vi "Initialization VI.vi"(8 "error in (no error)":errorcluster, 10 "Custom XML":string, 11 "Device Item Ref in":T1 format="%.0x") -> (0 "error out":errorcluster, 3 "Device Item Ref out":T1 format="%.0x")   [LabVIEW 2023, in "NI 272x Resistive Simulation Custom Device Configuration.lvlib"]
uses:
  NI 272x Resistive Simulation Custom Device Configuration.lvlib
  <vilib>/NI VeriStand/Custom Device API/Custom Device Item Ref.ctl
  <vilib>/NI VeriStand/Custom Device API/Custom Device Loop Type.ctl
  <vilib>/NI VeriStand/Custom Device API/Custom Device API.lvlib
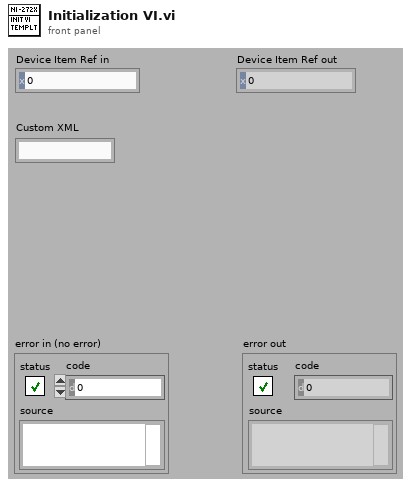
[diagram p1: front panel]
types:
  T1 = typedef "Custom Device API.lvlib/Custom Device Item Ref.ctl" = u64
  T2 = typedef "Custom Device API.lvlib/Custom Device Loop Type.ctl" = enum32{"While Loop", "Timed Loop"}
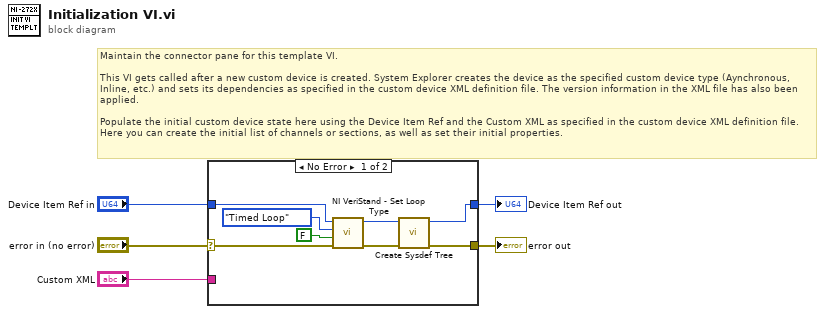
[diagram p0: block diagram]
diagram:
  # "Maintain the connector pane for this template VI.\n\nThis VI gets called after a new custom device is created. System Explorer creates the device as the specified custom device type (Aynchronous, Inline, etc.) and sets its dependencies as specified in the custom device XML definition file. The version information in the XML file has also been applied.\n\nPopulate the initial custom device state here using the Device Item Ref and the Custom XML as specified in the custom device XML definition file. Here you can create the initial list of channels or sections, as well as set their initial properties."
  n1 = case shown="No Error" "error in (no error)" {
    selector: "error in (no error)" -> [w13 w15]
    tunnel: [w9 w15] -> w5
    tunnel: [w8 w14] -> w3
    tunnel: "Device Item Ref in" -> [w12 w14]
    tunnel: "Custom XML" -> [_ _]
    frame No Error {
      n2 = call <vilib>:"NI VeriStand - Set Loop Type.vi"("error in (no error)"=w13, "Use Device Clock (Timed Loops only)"=FALSE, "Loop type"=Custom_Device_Loop_Type."Timed Loop", "Device Ref in"=w12) -> ("error out"=w6:errorcluster, "Device Ref out"=w7:T1)  [unwired: 6 in]
      n3 = call "Create Sysdef Tree.vi"("error in (no error)"=w6, "Device Ref"=w7) -> ("error out"=w9:errorcluster, "Device Ref Out"=w8:T1)  [unwired: 7 in]
    }
    frame Error {
    }
  }
  "error out" <- w5
  "Device Item Ref out" <- w3
